vi "Create Reply Sockets.vi"(8 "error in":errorcluster, 9 "Target Virt Instrs":T1(array[cluster]), 10 "Series Base in":refnum<class "Series Base.lvclass">, 11 "Study Actor in":refnum<class "Study Actor.lvclass">) -> (0 "error out":errorcluster, 3 "Study Actor out":refnum<class "Study Actor.lvclass">)   [LabVIEW 2023, in "Study Actor.lvlib" / "Study Actor.lvclass"]
uses:
  Study Actor.lvclass
  Series/Series Base/Series Base.lvclass
  Series/Series Base/Series Base.lvclass/Series Base.ctl
  Study Actor.lvclass/Study Actor.ctl
  Task/Task Base/Task Base.lvclass/Task Base.ctl
  Reply Protocol/Reply Protocol DataSocket/Reply Protocol DataSocket.lvclass
  D:/git/HAL/HAL GOOP4/Reply Protocol/Reply Protocol Base/Reply Protocol Base.lvclass
  Reply Protocol/Reply Protocol Base/Reply Protocol Base.lvclass/Reply Protocol Base.ctl
  Reply Protocol/Reply Protocol DataSocket/Reply Protocol DataSocket.lvclass/Reply Protocol DataSocket.ctl
  Task/Task Base/Task Base.lvclass
  Reply Protocol Manager/Reply Protocol Manager.lvclass
  Reply Protocol/Reply Protocol Base/Reply Protocol Base.lvclass
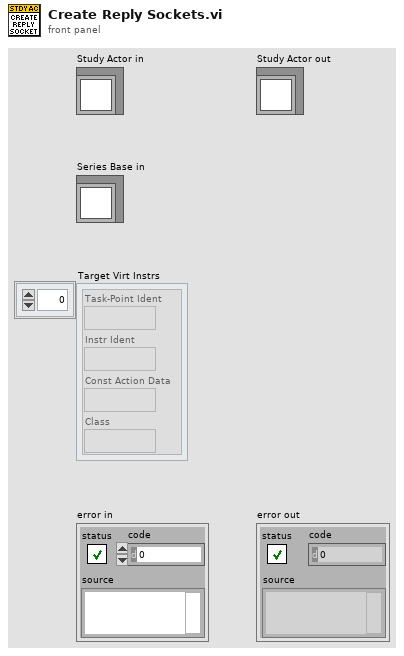
[diagram p1: front panel]
types:
  T1 = cluster{"Task-Point Ident":string, "Instr Ident":string, "Const Action Data":string, "Class":string}[]
  T2 = enum16{"Read", "Write", "ReadWrite", "BufferedRead", "BufferedReadWrite"}
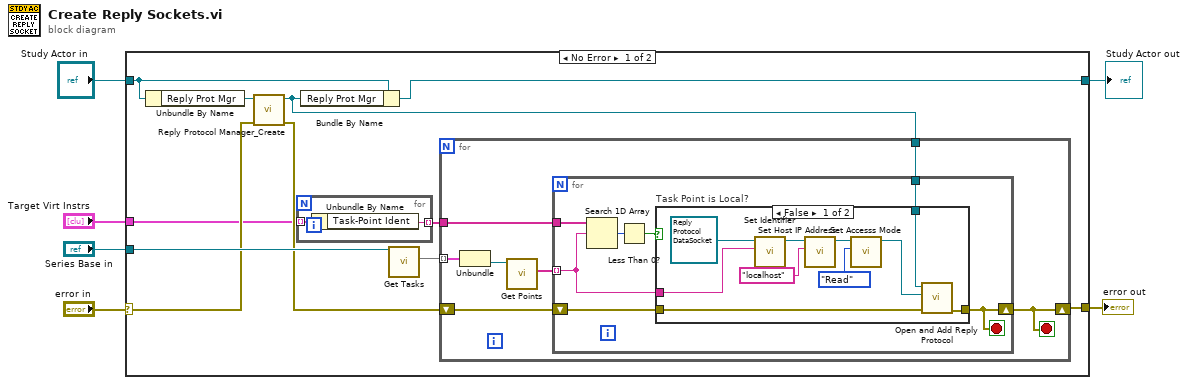
[diagram p0: block diagram]
diagram:
  n1 = case shown="No Error" "error in" {
    selector: "error in" -> [w14 w46]
    tunnel: [w15 w46] -> w5
    tunnel: [w10 w45] -> w3
    tunnel: "Study Actor in" -> [w11 w45]
    tunnel: "Series Base in" -> [w16 _]
    tunnel: "Target Virt Instrs" -> [w8 _]
    frame No Error {
      n2 = Unbundle By Name(w11) -> ("Reply Prot Mgr"=w12:refnum<class "Reply Protocol Manager.lvclass">)
      n3 = call "Reply Protocol Manager_Create.vi"("Error In"=w14, "reference in"=w12) -> ("Error Out"=w13:errorcluster, "reference out"=w9:refnum<class "Reply Protocol Manager.lvclass">)  [unwired: 8 in]
      n4 = for {
        tunnel: w8 -> [w19] mode=indexing
        tunnel: [w18] -> w7 mode=indexing
        n5 = Unbundle By Name(w19) -> ("Task-Point Ident"=w18:string)
      }
      n6 = Bundle By Name(cluster=w11, "Reply Prot Mgr"=w9) -> (w10:refnum<class "Study Actor.lvclass">)
      n7 = call "Get Tasks.vi"("HAL GOOP4:Series Base in"=w16) -> ("Tasks"=w17:map{string, refnum<class "Task Base.lvclass">})  [unwired: 9 in, 1 out]
      n8 = for {
        tunnel: w17 -> [w26] mode=indexing
        tunnel: w9 -> [w22]
        shift-right: [w21] -> w15
        shift-left: w13 -> [w23]
        tunnel: w7 -> [w20]
        stop <- w21 stop-if-true
        n9 = Unbundle(w26) -> ("Task"=w25:refnum<class "Task Base.lvclass">)  [unwired: 1 out]
        n10 = call "Get Points.vi"("Task Base in"=w25) -> ("Points"=w24:string[])  [unwired: 9 in, 1 out]
        n11 = for {
          tunnel: w20 -> [w33]
          tunnel: w24 -> [w31] mode=indexing
          tunnel: w22 -> [w28]
          shift-right: [w27] -> w21
          shift-left: w23 -> [w32]
          stop <- w27 stop-if-true
          n12 = Search 1D Array(1D array=w33, element=w31) -> (index of element=w30:i32)  [unwired: 1 in]
          n13 = Less Than 0?(x=w30) -> (x < 0?=w29:bool)
          n14 = case "Task Point is Local?" shown="False" w29 {
            tunnel: w32 -> [w40 w44]
            tunnel: [w39 w44] -> w27
            tunnel: w31 -> [w34 _]
            tunnel: w28 -> [w41 _]
            frame False {
              n15 = call "Set Identifier.vi"("Identifier"=w34, "Reply Protocol Base in"=refnum<class "Reply Protocol DataSocket.lvclass"> refnum ("HAL GOOP4.lvlib:Reply Protocol DataSocket.lvclass")) -> ("Reply Protocol Base out"=w43:refnum<class "Reply Protocol DataSocket.lvclass">)  [unwired: 9 in]
              n16 = call "Set Host IP Address.vi"("Host IP Address"="localhost", "Reply Protocol DataSocket in"=w43) -> ("Reply Protocol DataSocket out"=w38:refnum<class "Reply Protocol DataSocket.lvclass">)  [unwired: 9 in]
              n17 = call "Set Accesss Mode.vi"("Accesss Mode"=T2."Read", "Reply Protocol DataSocket in"=w38) -> ("Reply Protocol DataSocket out"=w36:refnum<class "Reply Protocol DataSocket.lvclass">)  [unwired: 9 in]
              n18 = call "Open and Add Reply Protocol.vi"("Error In"=w40, "Reply Protocol Base"=w36, "reference in"=w41) -> ("Error Out"=w39:errorcluster)  [unwired: 7 in, 1 out]
            }
            frame True {
            }
          }
        }
      }
    }
    frame Error {
    }
  }
  "error out" <- w5
  "Study Actor out" <- w3
